vi "Load.vi"(8 "error in (no error)":errorcluster, 10 "Path":path, 11 "Channel in":refnum<data-value>) -> (0 "error out":errorcluster, 3 "Channel out":refnum<data-value>)   [LabVIEW 2020, in "G-Audio.lvlib" / "Channel.lvclass"]
uses:
  Channel.lvclass
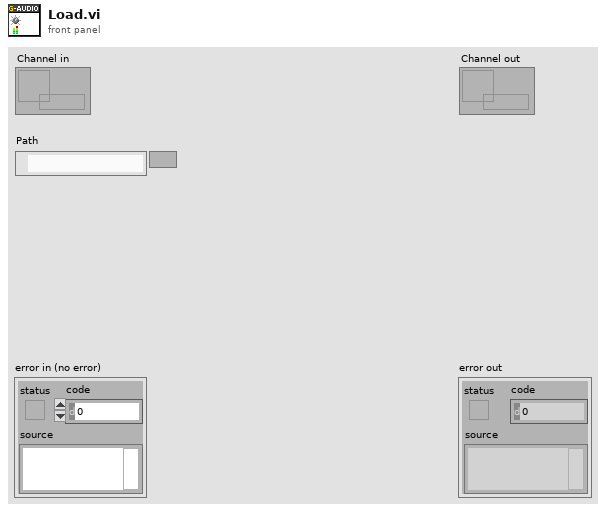
[diagram p1: front panel]
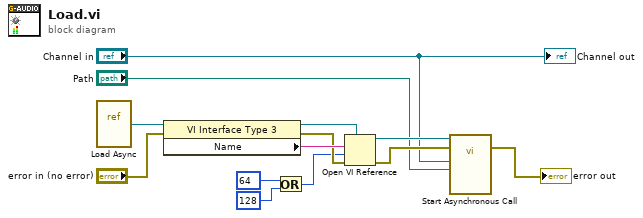
[diagram p0: block diagram]
diagram:
  n1 = vi-ref "Load Async.vi"() -> (w13:refnum<vi>)
  n2 = property class="VI Interface Type 3"(reference=w13, error in="error in (no error)") -> (reference out=w11:refnum<vi>, error out=w9:errorcluster, "Name"=w12:string)
  n3 = Or(x=64 ("options"), y=128 ("options")) -> (x .or. y?=w2:i32)
  n4 = Open VI Reference(type specifier VI Refnum (for type only)=w11, vi path=w12, options=w2, error in (no error)=w9) -> (vi reference=w10:refnum<vi>, error out=w8:errorcluster)  [unwired: 2 in]
  n5 = call-by-ref "Start Asynchronous Call"(reference=w10, error in=w8, "Path"="Path", "Channel in"="Channel in") -> (error out=→"error out":errorcluster)  [unwired: 8 in, 3 out]
  "Channel out" <- "Channel in"
